vi "motorTest.vi"() -> ()   [LabVIEW 2014]
uses:
  <vilib>/Rock Robotics/SystemInterfaces/Typedef/FPGA_TypedefDigitalModule.ctl
  <vilib>/Rock Robotics/SystemInterfaces/DIO/FPGA_DIOPWMChannel.ctl
  <vilib>/Rock Robotics/WPI/MotorControl/WPI_MotorControlOpen Victor.vi
panel:
  out "Motor Output":dbl
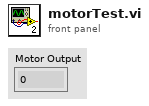
[diagram p1: front panel]
types:
  T1 = typedef "FPGA_DIOPWMChannel.ctl" = enum8{"PWM 0", "PWM 1", "PWM 2", "PWM 3", "PWM 4", "PWM 5", "PWM 6", "PWM 7", "PWM 8", "PWM 9", "PWM MXP 0", "PWM MXP 1", "PWM MXP 2", "PWM MXP 3", "PWM MXP 4", "PWM MXP 5", "PWM MXP 6", "PWM MXP 7", "PWM MXP 8", "PWM MXP 9", "Invalid"}
  T2 = typedef "FPGA_TypedefDigitalModule.ctl" = enum16{"Controller 1"}
  T3 = typedef "WPI_MotorControlDeviceRef.ctl" = cluster{"DeviceStatus":errorcluster, "Type":T4, "PWM":cluster{"Controller":T2, "PWM Channel":T1, "DeadBand":T5}, "CAN":cluster{"Device Number":u8, "Control Mode":T6, "Semaphore":T7, "Max Vout":dbl, "TalonSRX Control Mode":T8}, "Invert":bool, "TransformRef":T9, "InvTransformRef":T9}
  T4 = typedef "WPI_MotorControlType.ctl" = enum16{"PWM", "CAN", "CANTalonSRX"}
  T5 = typedef "WPI_PWMDeadband.ctl" = cluster{"Name":string, "maxPositivePwm":i32, "minPositivePwm":i32, "centerPwm":i32, "maxNegativePwm":i32, "minNegativePwm":i32, "angularRange":u16}
  T6 = typedef "WPI_CANJaguar_ControlMode.ctl" = enum8{"Percent VBus", "Current", "Speed", "Position", "Voltage"}
  T7 = typedef "Semaphore RefNum" = refnum<k1>
  T8 = typedef "WPI_CANTalonSRX_APIControlMode.ctl" = enum8{"Percent VBus", "Speed", "Position", "Slave", "Unchanged / Invalid"}
  T9 = typedef "WPI_PWMTransform_ConPane.ctl" = refnum<vi>
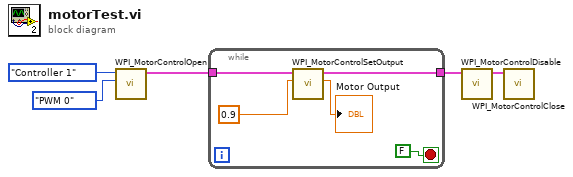
[diagram p0: block diagram]
diagram:
  n1 = call-poly <vilib>:"WPI_MotorControlOpen.vi"("PWM Channel"=FPGA_DIOPWMChannel."PWM 0", "Controller"=FPGA_TypedefDigitalModule."Controller 1") -> ("MotorControlDeviceRef"=w1:T3)  [unwired: 8 in, 1 out]
  n2 = while {
    tunnel: w1 -> [w10]
    tunnel: [w8] -> w3
    stop <- FALSE stop-if-true
    n3 = call <vilib>:"WPI_MotorControlSetOutput.vi"("Output"=0.9, "MotorControlDevRef"=w10) -> ("Motor Output"=→"Motor Output":dbl, "MotorControlDevRef"=w8:T3)  [unwired: 7 in, 1 out]
  }
  n4 = call <vilib>:"WPI_MotorControlDisable.vi"("MotorControlDevRef"=w3) -> ("MotorControlDevRef"=w2:T3)  [unwired: 9 in, 1 out]
  n5 = call <vilib>:"WPI_MotorControlClose.vi"("MotorControlDevRef"=w2) -> ()  [unwired: 10 in, 1 out]
